vi "LIN Slave Set ID Mode.vi"(6 "Len":u32, 7 "pLINMsg":T1, 9 "IDMode":u8, 10 "LINIndex":u8, 11 "DevHandle":i32) -> (3 "function return":i32, 5 "pLINMsg out":T1)   [LabVIEW 2010, in "USB2XXX.lvlib"]
doc: "int WINAPI LIN_SlaveSetIDMode(int DevHandle,unsigned char LINIndex,unsigned char IDMode,LIN_MSG *pLINMsg,unsigned int Len);"
uses:
  USB2XXX.lvlib
  USB2XXX.dll
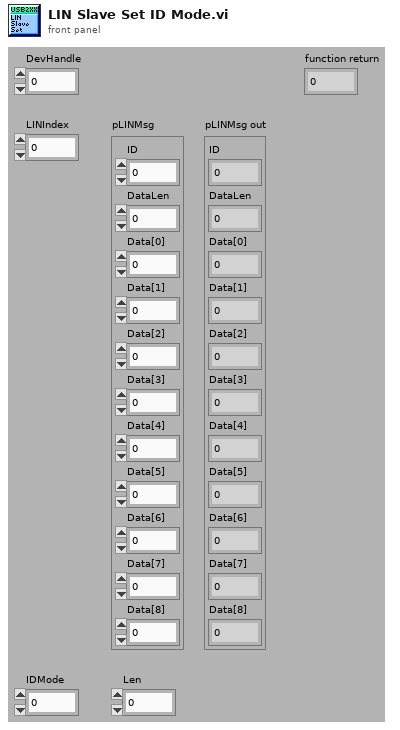
[diagram p1: front panel]
types:
  T1 = cluster{"ID":u8, "DataLen":u8, "Data[0]":u8, "Data[1]":u8, "Data[2]":u8, "Data[3]":u8, "Data[4]":u8, "Data[5]":u8, "Data[6]":u8, "Data[7]":u8, "Data[8]":u8}
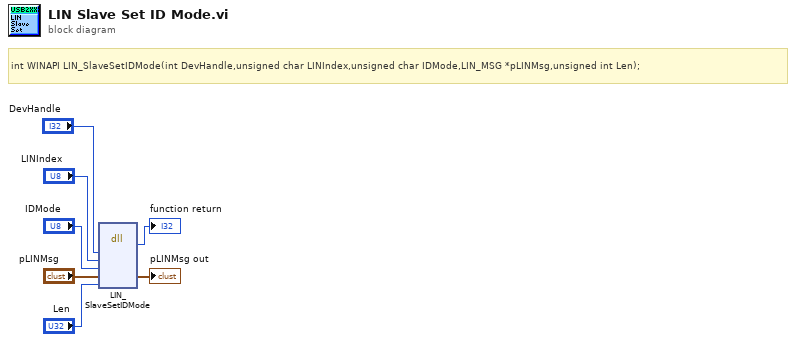
[diagram p0: block diagram]
diagram:
  # "int WINAPI LIN_SlaveSetIDMode(int DevHandle,unsigned char LINIndex,unsigned char IDMode,LIN_MSG *pLINMsg,unsigned int Len);"
  n1 = dll-call lib="F:/OtherWork/STM32/USB2XXX_Example/trunk/Labview/PublicFiles/USB2XXX.*" fn="LIN_SlaveSetIDMode"("DevHandle"="DevHandle", "LINIndex"="LINIndex", "IDMode"="IDMode", "pLINMsg"="pLINMsg", "Len"="Len") -> (→"function return":i32, "pLINMsg"=→"pLINMsg out":T1)  [unwired: 7 in, 2 out]
